vi "subDFD_Unset Busy VI.vi"(8 "error in (no error)":errorcluster, 11 "Busy vi reference":refnum<vi>) -> (0 "error out":errorcluster, 3 "dup Busy vi reference":refnum<vi>)   [LabVIEW 2017]
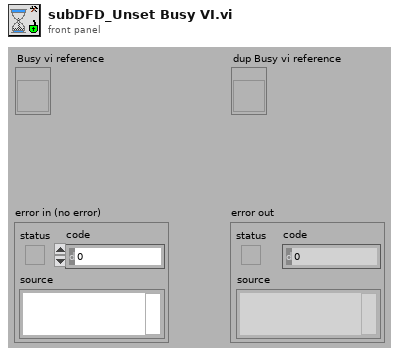
[diagram p1: front panel]
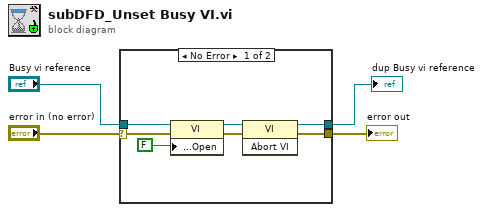
[diagram p0: block diagram]
diagram:
  n1 = case shown="No Error" "error in (no error)" {
    selector: "error in (no error)" -> [w5 w13]
    tunnel: "Busy vi reference" -> [w9 w12]
    tunnel: [w8 w12] -> w3
    tunnel: [w6 w13] -> w2
    frame No Error {
      n2 = property class="VI"(reference=w9, error in=w5, "Front Panel.Open"=FALSE ("Front Panel Window:Open")) -> (reference out=w10:refnum<vi>, error out=w7:errorcluster)
      n3 = invoke class="VI" method="Abort VI"(reference=w10, error in=w7) -> (reference out=w8:refnum<vi>, error out=w6:errorcluster)  [unwired: 1 in, 1 out]
    }
    frame Error {
    }
  }
  "dup Busy vi reference" <- w3
  "error out" <- w2
